vi "Render.vi"(11 "Main Controller Actor in":refnum<class "Main Controller Actor.lvclass">) -> (3 "Main Controller Actor out":refnum<class "Main Controller Actor.lvclass">)   [LabVIEW 2021, in "Main Controller Actor.lvclass"]
uses:
  Main Controller Actor.lvclass
  Main Controller Actor.lvclass/Main Controller Actor.ctl
  Galaxy/Galaxy.lvclass
  Element/Element.lvclass
  Renderer/Renderer.lvclass
  Globals.vi
  b0efc5d4-a195-4c67-8c97-309e47bb2d06.vi
  9709e86e-3adb-4b13-9239-b52712d00f61.vi
panel:
  out "Render Time [s]":dbl format="%.1p"
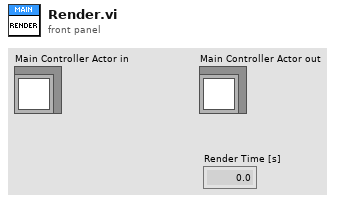
[diagram p1: front panel]
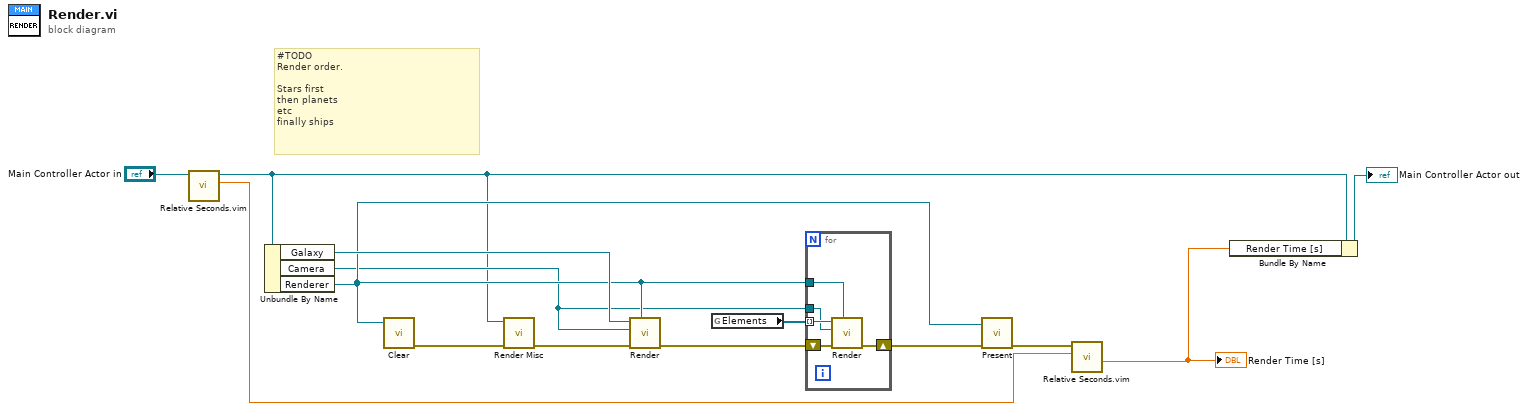
[diagram p0: block diagram]
diagram:
  # "#TODO\nRender order.\n\nStars first\nthen planets\netc\nfinally ships"
  n1 = call "Relative Seconds.vim"("Anything in"="Main Controller Actor in") -> ("Relative Seconds out"=w9:dbl, "Anything out"=w1:refnum<class "Main Controller Actor.lvclass">)  [unwired: 8 in, 1 out]
  n2 = Unbundle By Name(w1) -> ("Galaxy"=w7:refnum<class "Galaxy.lvclass">, "Camera"=w3:refnum<class "Camera.lvclass">, "Renderer"=w6:refnum<class "Renderer.lvclass">)
  n3 = call "Clear.vi"("Renderer"=w6) -> ("error out"=w12:errorcluster)  [unwired: 10 in]
  n4 = call "Render Misc.vi"("error in (no error)"=w12, "Main Controller Actor in"=w1) -> ("error out"=w5:errorcluster)  [unwired: 9 in]
  n5 = call-dynamic "Render.vi"("Renderer"=w6, "error in (no error)"=w5, "Camera"=w3, "Galaxy in"=w7) -> ("error out"=w4:errorcluster)  [unwired: 7 in]
  n6 = global read "Globals.vi" "Elements"() -> (w13:refnum<class "Element.lvclass">[])
  n7 = for {
    tunnel: w13 -> [w19] mode=indexing
    tunnel: w6 -> [w18]
    tunnel: w3 -> [w17]
    shift-right: [w15] -> w11
    shift-left: w4 -> [w16]
    n8 = call-dynamic "Render.vi"("Renderer"=w18, "error in (no error)"=w16, "Camera"=w17, "Element in"=w19) -> ("error out"=w15:errorcluster)  [unwired: 7 in]
  }
  n9 = call "Present.vi"("error in (no error)"=w11, "Renderer"=w6) -> ("error out"=w10:errorcluster)  [unwired: 9 in]
  n10 = call "Relative Seconds.vim"("Relative Seconds in"=w9, "Anything in"=w10) -> ("Relative Seconds delta"=w8:dbl)  [unwired: 7 in, 2 out]
  "Render Time [s]" <- w8
  n11 = Bundle By Name(cluster=w1, "Render Time [s]"=w8) -> (→"Main Controller Actor out":refnum<class "Main Controller Actor.lvclass">)
